vi "test6.2-RegisterInterruptFromNonCSM.vi"(8 "error in (no error)":errorcluster, 11 "TestCase in":refnum<class "testcase-CSMBroadcast.lvclass">) -> (0 "error out":errorcluster, 3 "TestCase out":refnum<class "testcase-CSMBroadcast.lvclass">)   [LabVIEW 2017, in "testcase-CSMBroadcast.lvclass"]
uses:
  testcase-CSMBroadcast.lvclass
  <vilib>/addons/_JKI Toolkits/VI Tester/TestCase.llb/TestCase.lvclass
  src/user.lib/_NEVSTOP/Communicable State Machine(CSM)/Communicable State Machine.lvlib
  C:/Program Files (x86)/National Instruments/LabVIEW 2017/vi.lib/addons/_JKI Toolkits/VI Tester/TestCase.llb/TestCase.lvclass
panel:
  out "output cluster":T1
  out "error out 3":errorcluster
  out "error out 2":errorcluster
  out "LoopCount":i32
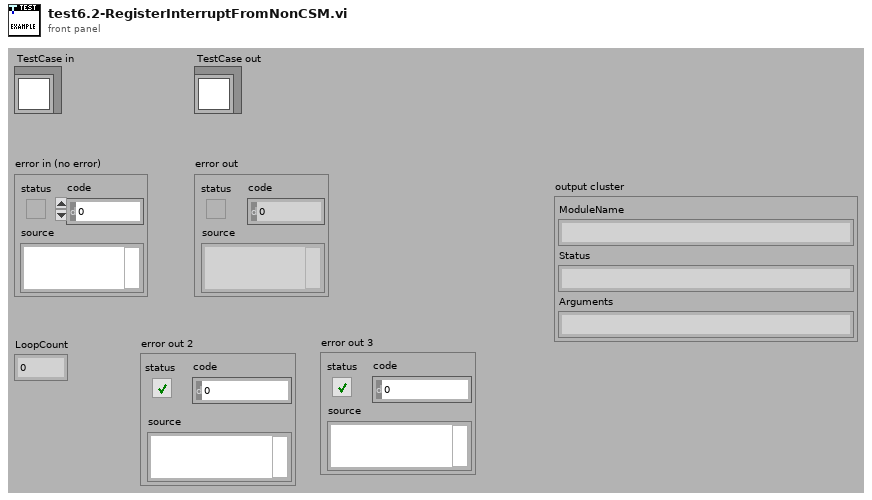
[diagram p1: front panel]
types:
  T1 = cluster{"ModuleName":string, "Status":string, "Arguments":string}
  T2 = cluster{"Status Event":refnum<user-event>, "Interrupt Event":refnum<user-event>}
  T3 = cluster{"cluster":cluster{"ModuleName":string, "Status":string, "Arguments":string}}
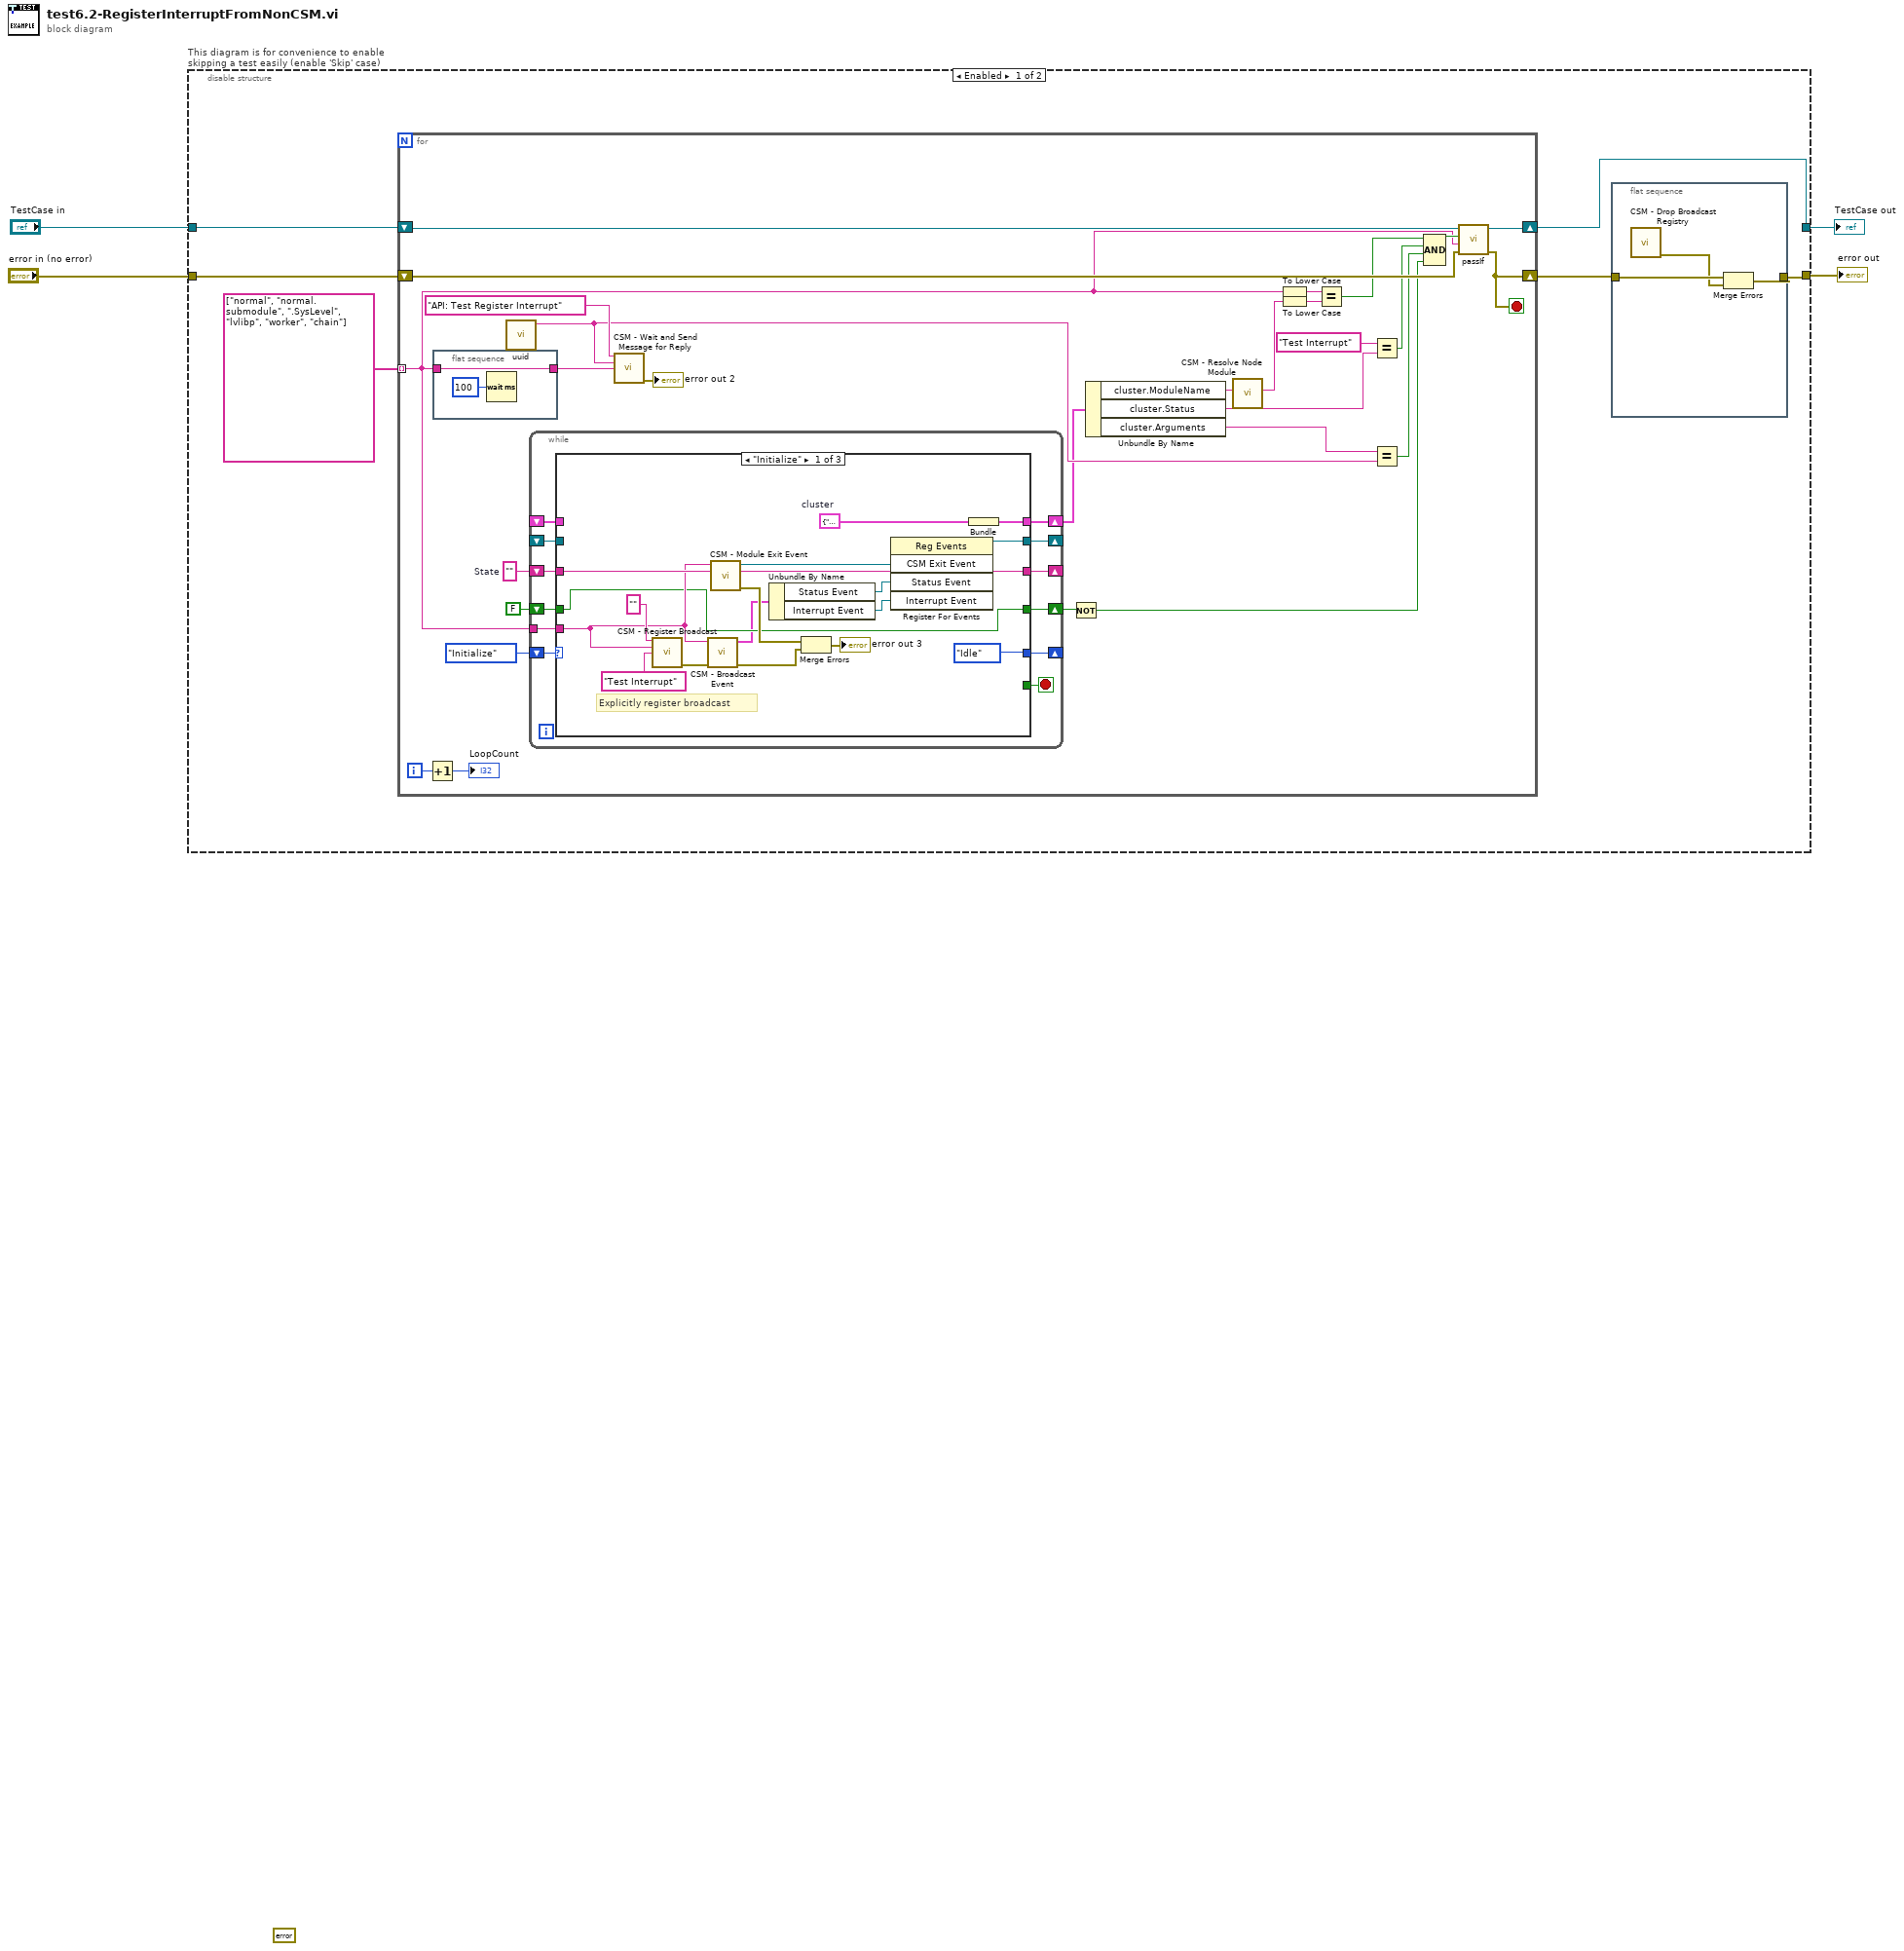
[diagram p0: block diagram]
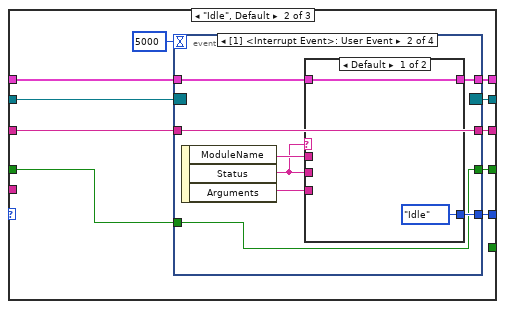
[diagram p2: hidden frame]
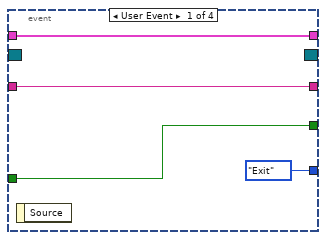
[diagram p3: hidden frame]
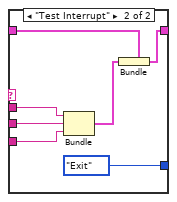
[diagram p4: hidden frame]
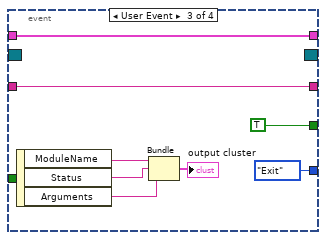
[diagram p5: hidden frame]
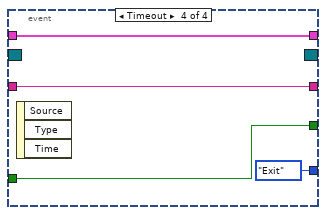
[diagram p6: hidden frame]
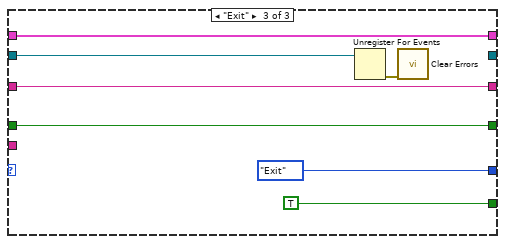
[diagram p7: hidden frame]
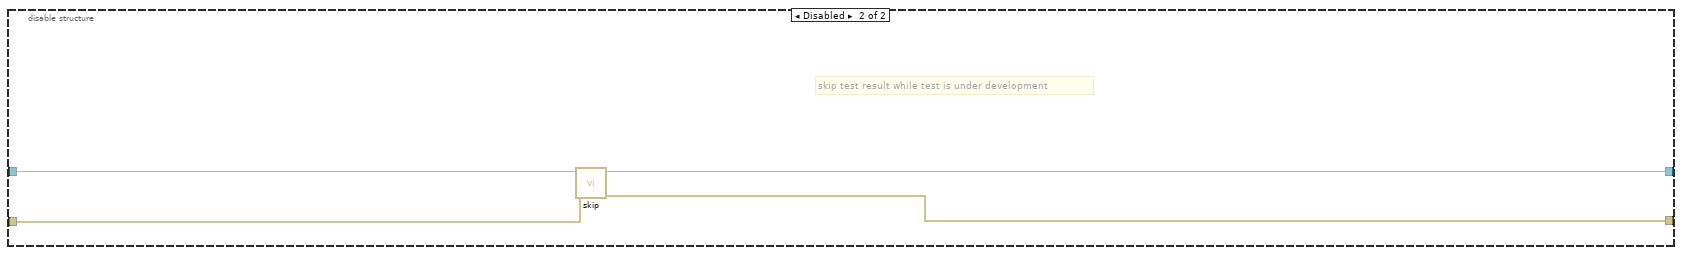
[diagram p8: hidden frame]
diagram:
  (unwired) errorcluster {"status"=FALSE, "code"=0, "source"=""} ("error out")
  n1 = disable-structure "This diagram is for convenience to enable skipping a test easily (enable 'Skip' case)" shown="Enabled" {
    disable-tunnel: "TestCase in" -> [w10 w126]
    disable-tunnel: [w6 w124] -> w2
    disable-tunnel: [w5 w125] -> w1
    disable-tunnel: "error in (no error)" -> [w9 w123]
    frame Enabled {
      n2 = for {
        shift-right: [w32] -> w6
        shift-left: w10 -> [w33]
        tunnel: string[] ["normal", "normal.submodule", ".SysLevel", "lvlibp", "worker", "chain"] -> [w18] mode=indexing
        shift-right: [w23] -> w7
        shift-left: w9 -> [w31]
        i -> [w26]
        stop <- w23 stop-if-true
        w40 = ""  # State
        n3 = Increment(x=w26) -> (x+1=→"LoopCount":i32)
        n4 = flat-sequence {
          tunnel: w18 -> [w43]
          tunnel: [w43] -> w38
          frame #0 {
            n5 = Wait (ms)(milliseconds to wait=u32 100) -> ()  [unwired: 1 out]
          }
        }
        n6 = call "uuid.vi"() -> ("UUID"=w35:string)  [unwired: 11 in]
        n7 = while {
          shift-right: [w54] -> _
          shift-left: enum16{"Idle", "Initialize", "Exit"}."Initialize" -> [w55]
          shift-right: [w51] -> _
          shift-left: w40 -> [w52]
          shift-right: [w50] -> _
          shift-left: _ -> [w49]
          shift-right: [w48] -> w22
          shift-left: _ -> [w47]
          tunnel: w18 -> [w46]
          shift-right: [w45] -> w16
          shift-left: FALSE -> [w44]
          stop <- w53 stop-if-true
          n8 = case shown="\"Initialize\"" w55 {
            tunnel: [enum16{"Idle", "Initialize", "Exit"}."Idle" w82 enum16{"Idle", "Initialize", "Exit"}."Exit"] -> w54
            tunnel: [_ _ TRUE] -> w53
            tunnel: w52 -> [w71 w80 w120]
            tunnel: [w71 w81 w120] -> w51
            tunnel: [w69 w78 _] -> w50
            tunnel: w49 -> [_ w79 w119]
            tunnel: [w68 w76 w117] -> w48
            tunnel: w47 -> [_ w77 w117]
            tunnel: w46 -> [w60 _ _]
            tunnel: [w57 w74 w116] -> w45
            tunnel: w44 -> [w57 w73 w116]
            frame "Initialize" {
              w67 = T1 {"ModuleName"="", "Status"="", "Arguments"=""}  # cluster
              # "Explicitly register broadcast"
              n9 = call "CSM - Register Broadcast.vi"("CSM Name(Empty for Broadcast Event)"="", "Source CSM Name (* as Default)"=w60, "Trigger"="Test Interrupt" ("State")) -> ("error out"=w62:errorcluster)  [unwired: 11 in, 1 out]
              n10 = call "CSM - Broadcast Event.vi"("Error In"=w62, "CSM Module"=w60) -> ("error out"=w65:errorcluster, "Broadcast Event"=w56:T2)  [unwired: 7 in, 1 out]
              n11 = call "CSM - Module Exit Event.vi"("Name (\"\" to Use UUID) In"=w60) -> ("error out"=w66:errorcluster, "CSM Exit Event"=w70:refnum<user-event>)  [unwired: 8 in, 1 out]
              n12 = Unbundle By Name(w56) -> ("Status Event"=w59:refnum<user-event>, "Interrupt Event"=w58:refnum<user-event>)
              n13 = Merge Errors(w66, w65) -> (→"error out 3":errorcluster)
              n14 = register-events(w70, w59, w58) -> (reference out=w69:refnum<event-registration>)  [unwired: 2 in, 1 out]
              n15 = Bundle("cluster"=w67) -> (w68:T3)  [unwired: 1 in]
            }
            frame "Idle", Default {
              n16 = event shown="[1] <Interrupt Event>: User Event" {
                selector: w79 -> [_ _ _ _]
                dyn-events: [_ _ _ _] -> w78
                timeout: 5000 -> [_ _ _ _]
                tunnel: [enum16{"Idle", "Initialize", "Exit"}."Exit" w93 enum16{"Idle", "Initialize", "Exit"}."Exit" enum16{"Idle", "Initialize", "Exit"}."Exit"] -> w82
                tunnel: w80 -> [w86 w94 w111 w115]
                tunnel: [w86 w94 w111 w115] -> w81
                tunnel: w77 -> [w84 w90 w110 w114]
                tunnel: [w84 w89 w110 w114] -> w76
                tunnel: [w83 w87 TRUE w112] -> w74
                tunnel: w73 -> [w83 w87 _ w112]
                event User Event {
                  n17 = event-data() -> ()  [unwired: 1 in, 1 out]
                }
                event User Event {
                  n18 = event-data() -> ("ModuleName"=w92:string, "Status"=w88:string, "Arguments"=w91:string)  [unwired: 1 in]
                  n19 = case shown="Default" w88 {
                    tunnel: [enum16{"Idle", "Initialize", "Exit"}."Idle" enum16{"Idle", "Initialize", "Exit"}."Exit"] -> w93
                    tunnel: w92 -> [_ w102]
                    tunnel: w88 -> [_ w101]
                    tunnel: w91 -> [_ w100]
                    tunnel: w90 -> [w96 w99]
                    tunnel: [w96 w97] -> w89
                    frame Default {
                    }
                    frame "Test Interrupt" {
                      n20 = Bundle("ModuleName"=w102, "Status"=w101, "Arguments"=w100) -> (w98:T1)  [unwired: 1 in]
                      n21 = Bundle(cluster=w99, "cluster"=w98) -> (w97:T3)
                    }
                  }
                }
                event User Event {
                  n22 = event-data() -> ("ModuleName"=w107:string, "Status"=w106:string, "Arguments"=w105:string)  [unwired: 1 in]
                  n23 = Bundle("ModuleName"=w107, "Status"=w106, "Arguments"=w105) -> (→"output cluster":T1)  [unwired: 1 in]
                }
                event Timeout {
                  n24 = event-data() -> ()  [unwired: 1 in, 3 out]
                }
              }
            }
            frame "Exit" {
              n25 = Unregister For Events(event registration refnum=w119) -> (error out=w118:errorcluster)  [unwired: 1 in]
              n26 = call <vilib>:"Clear Errors.vi"("error in (no error)"=w118) -> ()  [unwired: 5 in, 2 out]
            }
          }
        }
        n27 = call "CSM - Wait and Send Message for Reply.vi"("State"="API: Test Register Interrupt", "Arguments (\"\")"=w35, "Target Module"=w38) -> ("error out"=→"error out 2":errorcluster)  [unwired: 10 in, 2 out]
        n28 = Not(x=w16) -> (.not. x?=w15:bool)
        n29 = Unbundle By Name(w22) -> ("cluster.ModuleName"=w20:string, "cluster.Status"=w36:string, "cluster.Arguments"=w34:string)
        n30 = call "CSM - Resolve Node Module.vi"("Node Name"=w20) -> ("CSM Module Name"=w17:string)  [unwired: 10 in]
        n31 = To Lower Case(string=w18) -> (all lower case string=w21:string)
        n32 = To Lower Case(string=w17) -> (all lower case string=w19:string)
        n33 = Equal?(x=w21, y=w19) -> (x = y?=w30:bool)
        n34 = Equal?(x="Test Interrupt" ("State"), y=w36) -> (x = y?=w29:bool)
        n35 = Equal?(x=w34, y=w35) -> (x = y?=w28:bool)
        n36 = Compound Arithmetic op=AND(w30, w29, w28, w15) -> (w27:bool)
        n37 = call-dynamic "passIf.vi"("error in (no error)"=w31, "message (\"\")"=w18, "pass"=w27, "TestCase in"=w33) -> ("error out"=w23:errorcluster, "TestCase out"=w32:refnum<class "testcase-CSMBroadcast.lvclass">)  [unwired: 6 in]
      }
      n38 = flat-sequence {
        tunnel: w7 -> [w13]
        tunnel: [w12] -> w5
        frame #0 {
          n39 = call "CSM - Drop Broadcast Registry.vi"() -> ("error out"=w11:errorcluster)  [unwired: 15 in]
          n40 = Merge Errors(w13, w11) -> (w12:errorcluster)
        }
      }
    }
    frame Disabled {
      # "skip test result while test is under development"
      n41 = call <vilib>:"skip.vi"("error in (no error)"=w123, "TestCase in"=w126) -> ("error out"=w125:errorcluster, "TestCase out"=w124:refnum<class "testcase-CSMBroadcast.lvclass">)  [unwired: 8 in]
    }
  }
  "error out" <- w1
  "TestCase out" <- w2
